vi "Show.vi"(11 "Picture in":refnum<class "Picture.lvclass">) -> (1 "Pixmap 2D":u32[][](array[numeric]), 3 "Picture out":refnum<class "Picture.lvclass">)   [LabVIEW 2018]
uses:
  Picture.lvclass
  Picture.lvclass/Picture.ctl
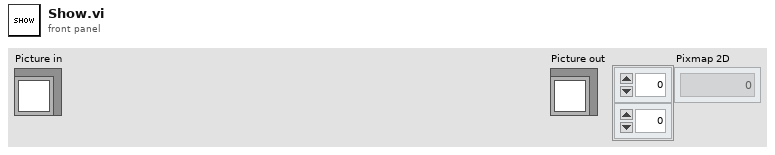
[diagram p1: front panel]
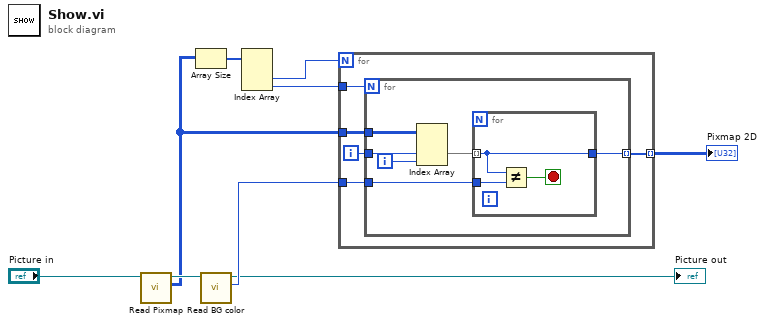
[diagram p0: block diagram]
diagram:
  n1 = call "Read Pixmap.vi"("Picture in"="Picture in") -> ("3D Pixmap"=w5:u32[][][], "Picture out"=w8:refnum<class "Picture.lvclass">)  [unwired: 8 in, 1 out]
  n2 = Array Size(array=w5) -> (size(s)=w9:i32[])
  n3 = call "Read BG color.vi"("Picture in"=w8) -> ("BG color"=w4:u32, "Picture out"=→"Picture out":refnum<class "Picture.lvclass">)  [unwired: 8 in, 1 out]
  n4 = Index Array(array=w9) -> (element #2=w7:i32, element #3=w6:i32)  [unwired: 3 in, 1 out]
  n5 = for {
    N: w7 -> [_]
    tunnel: w6 -> [w14]
    tunnel: w5 -> [w13]
    tunnel: w4 -> [w11]
    tunnel: [w10] -> w2 mode=indexing
    i -> [w12]
    n6 = for {
      N: w14 -> [_]
      tunnel: w13 -> [w20]
      tunnel: w12 -> [w19]
      tunnel: w11 -> [w16]
      tunnel: [w15] -> w10 mode=indexing
      i -> [w18]
      n7 = Index Array(array=w20, index (dim 1)=w19, index (dim 2)=w18) -> (element=w17:u32[])  [unwired: 1 in]
      n8 = for {
        tunnel: w17 -> [w21] mode=indexing
        tunnel: w16 -> [w23]
        tunnel: [w21] -> w15
        stop <- w22 stop-if-true
        n9 = Not Equal?(x=w21, y=w23) -> (x != y?=w22:bool)
      }
    }
  }
  "Pixmap 2D" <- w2
